vi "Untitled 10.vi"() -> ()   [LabVIEW 2023]
panel:
  out "Licznik":i32
  in  "Reset/Count":bool
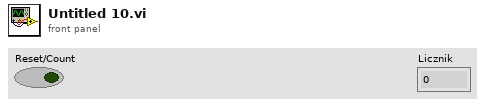
[diagram p1: front panel]
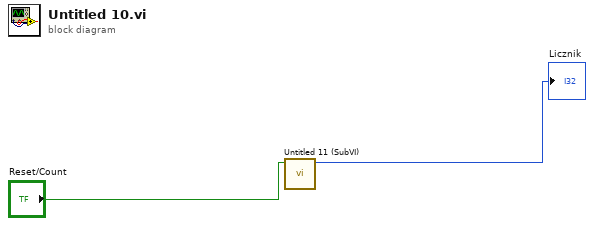
[diagram p0: block diagram]
diagram:
  n1 = call "Untitled 11 (SubVI).vi"("Reset/Count"="Reset/Count") -> ("f"=→"Licznik":i32)  [unwired: 10 in]
